vi "Query Generator ARB File Path.vi"(8 "error in (no error)":errorcluster, 9 "Type (Relative)":i32(ring) items=["Relative", "Absolute"], 10 "Instance (1)":i32=1, 11 "VISA resource name":refnum<visa-resource-name>) -> (0 "error out":errorcluster, 2 "File Path":string, 3 "VISA resource name out":refnum<visa-resource-name>)   [LabVIEW 2020, in "Rohde&Schwarz CMXP GPRF.lvlib"]
doc: "Queries the path of the loaded waveform file.\n\nAttributes:\nRSCMXPGPRF_ATTR_ARB_FILE\nRSCMXPGPRF_ATTR_ARB_GET_FILE_ABS_PATH\n\nRemote-control commands:\nSOURce:GPRF:GEN<i>:ARB:FILE\nSOURce:GPRF:GEN<i>:ARB:FILE?"
uses:
  <instrlib>/Rohde&Schwarz CMXP GPRF/Rohde&Schwarz CMXP GPRF.lvlib
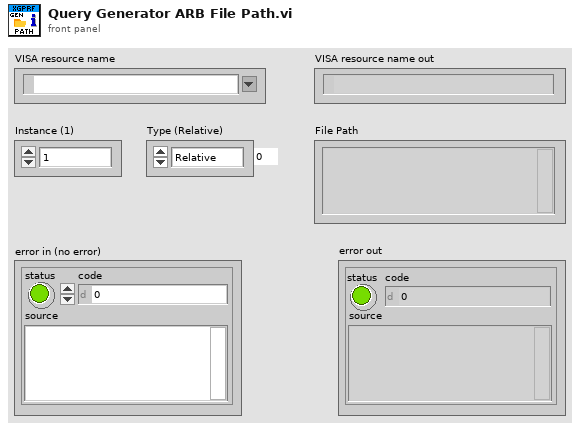
[diagram p1: front panel]
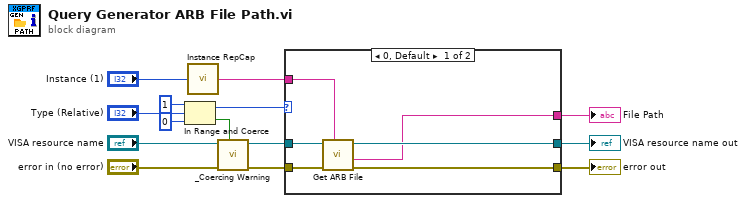
[diagram p0: block diagram]
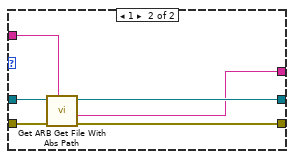
[diagram p2: hidden frame]
diagram:
  n1 = In Range and Coerce(upper limit=1, x="Type (Relative)", lower limit=0) -> (coerced(x)=w5:i32, In Range?=w4:bool)
  n2 = call <instrlib>:"Instance RepCap.vi"("Instance in"="Instance (1)") -> ("Instance out"=w14:string)
  n3 = call <instrlib>:"_Coercing Warning.vi"("In Range?"=w4, "error in (no error)"="error in (no error)", "VISA resource name"="VISA resource name") -> ("error out"=w10:errorcluster, "VISA resource name out"=w9:refnum<visa-resource-name>)  [unwired: 7 in]
  n4 = case shown="0, Default" w5 {
    tunnel: w14 -> [w20 w26]
    tunnel: w9 -> [w19 w25]
    tunnel: w10 -> [w18 w24]
    tunnel: [w17 w23] -> w2
    tunnel: [w16 w22] -> w3
    tunnel: [w15 w21] -> w1
    frame 0, Default {
      n5 = call "Get ARB File"("Repeated Capabilities"=w20, "error in (no error)"=w18, "instrument handle"=w19) -> ("error out"=w16:errorcluster, "ARB File"=w15:string, "instrument handle out"=w17:refnum<visa-resource-name>)  [unwired: 6 in]
    }
    frame 1 {
      n6 = call "Get ARB Get File With Abs Path"("Repeated Capabilities"=w26, "error in (no error)"=w24, "instrument handle"=w25) -> ("error out"=w22:errorcluster, "ARB Get File With Abs Path"=w21:string, "instrument handle out"=w23:refnum<visa-resource-name>)  [unwired: 6 in]
    }
  }
  "error out" <- w3
  "VISA resource name out" <- w2
  "File Path" <- w1
